vi "3D_Session_Data.vi"(10 "Session":i32) -> (1 "Radius":sgl, 2 "min":dbl, 3 "max":dbl)   [LabVIEW 2011]
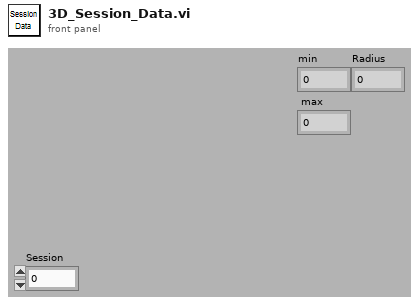
[diagram p1: front panel]
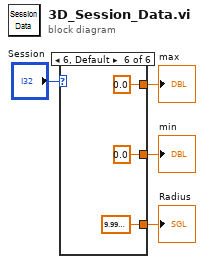
[diagram p0: block diagram]
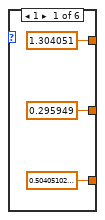
[diagram p2: hidden frame]
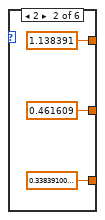
[diagram p3: hidden frame]
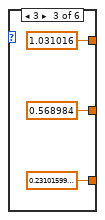
[diagram p4: hidden frame]
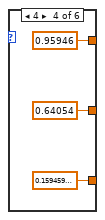
[diagram p5: hidden frame]
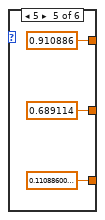
[diagram p6: hidden frame]
diagram:
  n1 = case shown="6, Default" "Session" {
    tunnel: [0.295949 ("y") 0.461609 ("y") 0.568984 ("y") 0.64054 ("y") 0.689114 ("y") 0.0 ("y")] -> w1
    tunnel: [1.304051 ("y") 1.138391 ("y") 1.031016 ("y") 0.95946 ("y") 0.910886 ("y") 0.0 ("y")] -> w2
    tunnel: [sgl 0.504051 ("Radius") sgl 0.338391 ("Radius") sgl 0.231016 ("Radius") sgl 0.15946 ("Radius") sgl 0.110886 ("Radius") sgl 0.0001 ("Radius")] -> w3
    frame 1 {
    }
    frame 2 {
    }
    frame 3 {
    }
    frame 4 {
    }
    frame 5 {
    }
    frame 6, Default {
    }
  }
  "min" <- w1
  "max" <- w2
  "Radius" <- w3
